vi "close.vi"(8 "error in (no error)":errorcluster, 11 "PSP-603 in":refnum<class "PSP-603.lvclass">) -> (0 "error out":errorcluster, 3 "PSP-603 out":refnum<class "PSP-603.lvclass">)   [LabVIEW 2025, in "Power Supply.lvlib" / "PSP-603.lvclass"]
uses:
  PSP-603.lvclass
  PSP-603.lvclass/PSP-603.ctl
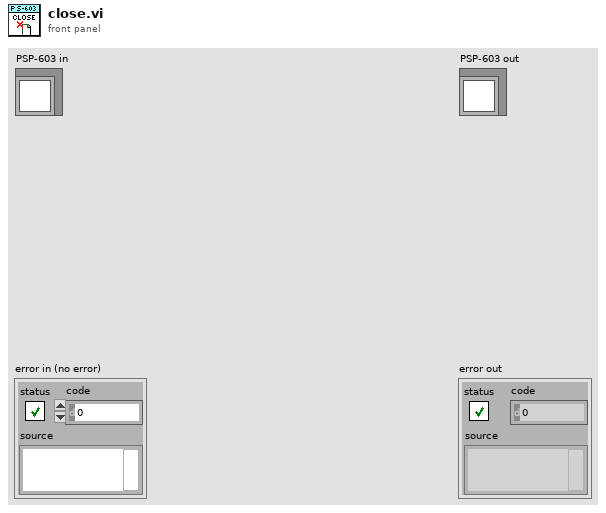
[diagram p1: front panel]
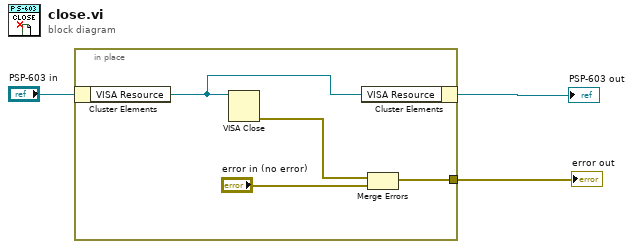
[diagram p0: block diagram]
diagram:
  n1 = in-place {
    in-place-border: [w4] -> w1
    n2 = in-place-cluster #1("PSP-603 in") -> ("VISA Resource"=w7:refnum<visa-resource-name>)
    n3 = VISA Close(VISA resource name=w7) -> (error out=w5:errorcluster)  [unwired: 1 in]
    n4 = in-place-cluster #1("VISA Resource"=w7) -> (→"PSP-603 out":refnum<class "PSP-603.lvclass">)
    n5 = Merge Errors(w5, "error in (no error)") -> (w4:errorcluster)
  }
  "error out" <- w1
